vi "StingDateToYesterday.vi"(8 "Days":dbl=1.0, 10 "Date":string="2014/10/01") -> (1 "Date-1 string":string, 3 "Date+1":string)   [LabVIEW 2012]
uses:
  <vilib>/Utility/miscctls.llb/LVDateTimeRec.ctl
panel:
  in  "date time rec":T1
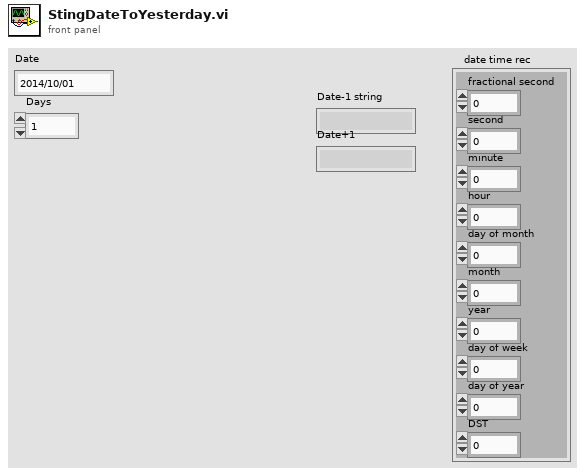
[diagram p1: front panel]
types:
  T1 = typedef "LVDateTimeRec.ctl" = cluster{"fractional second":dbl, "second":i32, "minute":i32, "hour":i32, "day of month":i32, "month":i32, "year":i32, "day of week":i32, "day of year":i32, "DST":i32}
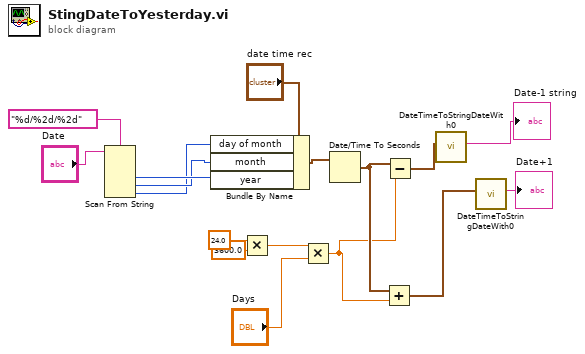
[diagram p0: block diagram]
diagram:
  n1 = Scan From String(format string="%d/%2d/%2d", input string="Date") -> (output 1=w14:i32, output 2=w13:i32, output 3=w12:i32)  [unwired: 5 in, 3 out]
  n2 = Bundle By Name(cluster="date time rec", "day of month"=w12, "month"=w13, "year"=w14) -> (w11:T1)
  n3 = Multiply(x=24.0, y=3600.0) -> (x*y=w8:dbl)
  n4 = Multiply(x=w8, y="Days") -> (x*y=w3:dbl)
  n5 = Date/Time To Seconds(2:w11) -> (0:w4:timestamp)  [unwired: 1 in]
  n6 = Add(x=w4, y=w3) -> (x+y=w6:timestamp)
  n7 = Subtract(x=w4, y=w3) -> (x-y=w2:timestamp)
  n8 = call "DateTimeToStringDateWith0.vi"("time stamp"=w2) -> ("String Date With0"=→"Date-1 string":string)  [unwired: 9 in, 1 out]
  n9 = call "DateTimeToStringDateWith0.vi"("time stamp"=w6) -> ("String Date With0"=→"Date+1":string)  [unwired: 9 in, 1 out]
